vi "Thermocouple_Volts to Temperature.vi"(5 "Temperature Units":u16(ring) items=["Celsius", "Fahrenheit", "Kelvin", "Rankine"], 6 "ThermocoupleType":u16(ring)=2 items=["B", "E", "J", "K", "R", "S", "T", "N"], 7 "Thermocouple Voltage":sgl format="%.6f") -> (3 "Temperature":sgl format="%.6f")   [LabVIEW 2019]
doc: "Converts a voltage read from a thermocouple into a temperature.\n\nNational Instruments has chosen thermocouple polynomial expressions that are valid only for particular temperature ranges (given in the VI diagram). These polynomials come from the NIST Monograph 175.\n\nIf you wish to use a different conversion formula, you can edit this VI and enter your own equation into the appropriate formula node."
panel:
  # "Convert a thermocouple voltage\nto temperature."
  # "National Instruments has chosen thermocouple polynomial expressions that are valid only for  particular temperature ranges (given in the VI diagram).  These polynomials come from the NIST Monograph 175.\n\nIf you wish to use a different conversion formula, you can edit this VI and enter your own equation into the appropriate formula node."
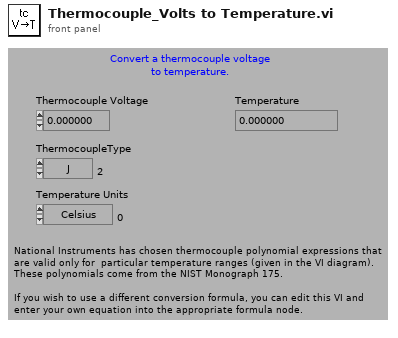
[diagram p1: front panel]
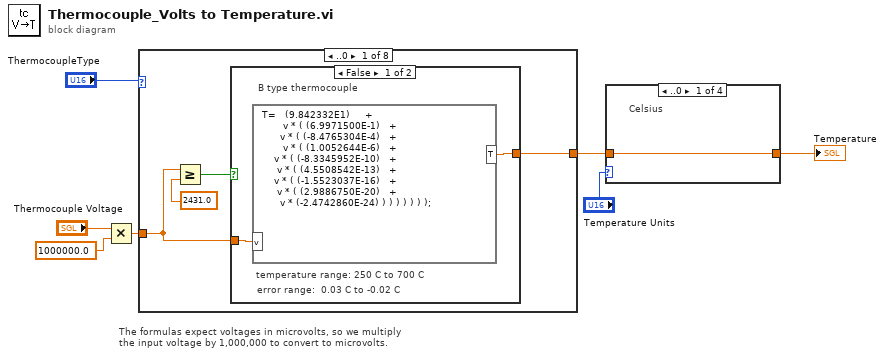
[diagram p0: block diagram]
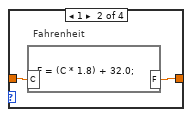
[diagram p2: hidden frame]
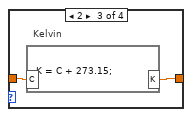
[diagram p3: hidden frame]
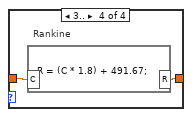
[diagram p4: hidden frame]
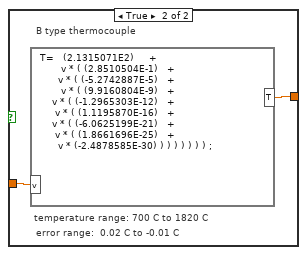
[diagram p5: hidden frame]
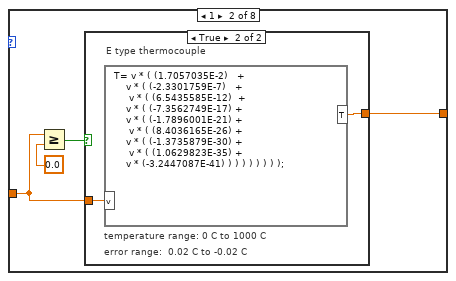
[diagram p6: hidden frame]
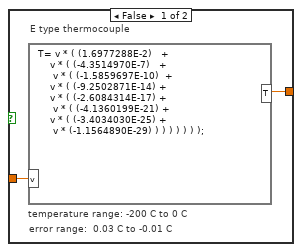
[diagram p7: hidden frame]
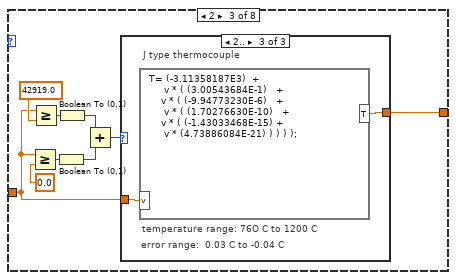
[diagram p8: hidden frame]
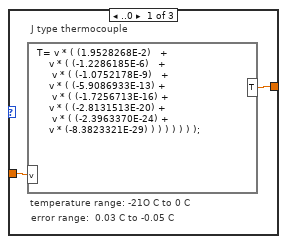
[diagram p9: hidden frame]
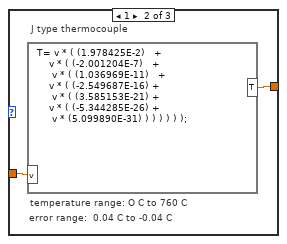
[diagram p10: hidden frame]
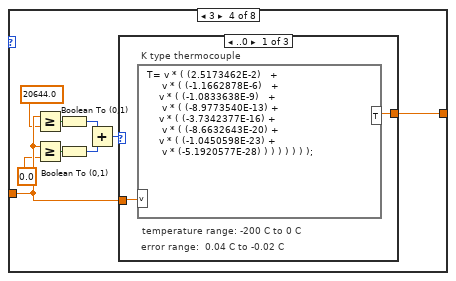
[diagram p11: hidden frame]
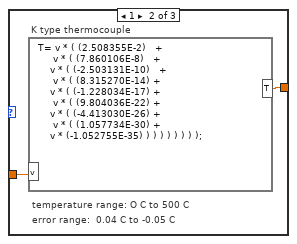
[diagram p12: hidden frame]
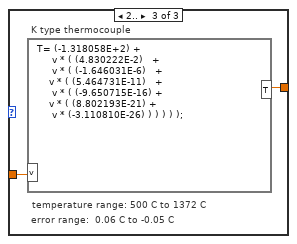
[diagram p13: hidden frame]
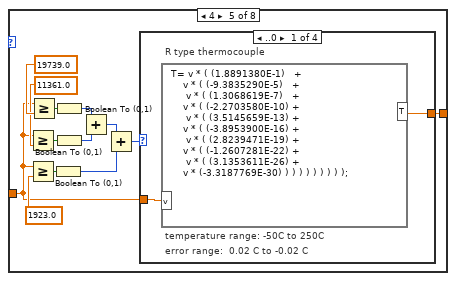
[diagram p14: hidden frame]
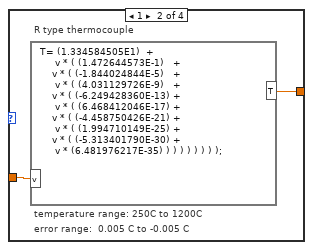
[diagram p15: hidden frame]
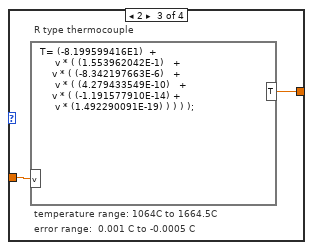
[diagram p16: hidden frame]
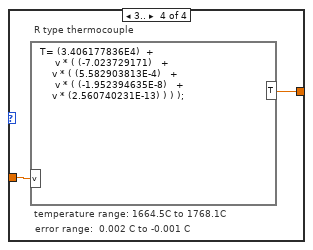
[diagram p17: hidden frame]
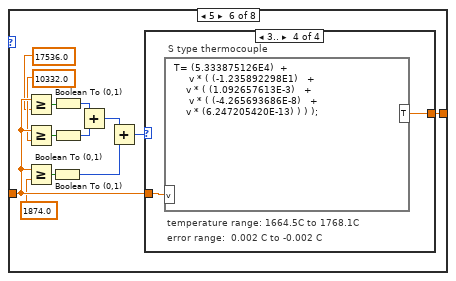
[diagram p18: hidden frame]
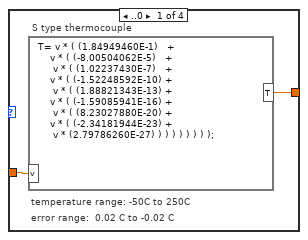
[diagram p19: hidden frame]
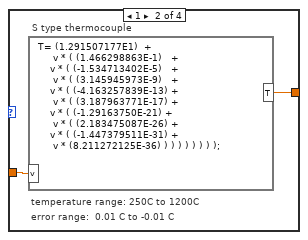
[diagram p20: hidden frame]
diagram:
  # "The formulas expect voltages in microvolts, so we multiply\nthe input voltage by 1,000,000 to convert to microvolts."
  n1 = Multiply(x="Thermocouple Voltage", y=sgl 1000000.0) -> (x*y=w4:sgl)
  n2 = case shown="..0" "ThermocoupleType" {
    tunnel: [w11 w18 w32 w39 w66 w87 w99 w111] -> w2
    tunnel: w4 -> [w9 w16 w24 w47 w54 w83 w96 w110]
    frame ..0 {
      n3 = Greater Or Equal?(x=w9, y=sgl 2431.0) -> (x >= y?=w10:bool)
      n4 = case shown="False" w10 {
        tunnel: w9 -> [w13 w15]
        tunnel: [w12 w14] -> w11
        frame False {
          # "error range:  0.03 C to -0.02 C"
          # "temperature range: 250 C to 700 C"
          # "B type thermocouple"
          n5 = formula code="T=   (9.842332E1)     +\n       v * ( (6.9971500E-1)   +\n      v * ( (-8.4765304E-4)   +\n       v * ( (1.0052644E-6)   +\n    v * ( (-8.3345952E-10)   +\n     v * ( (4.5508542E-13)   +\n    v * ( (-1.5523037E-16)   +\n     v * ( (2.9886750E-20)   +               \n      v * (-2.4742860E-24) ) ) ) ) ) ) );"("v"=w13) -> ("T"=w12:dbl)
        }
        frame True {
          # "error range:  0.02 C to -0.01 C"
          # "temperature range: 700 C to 1820 C"
          # "B type thermocouple"
          n6 = formula code="T=   (2.1315071E2)     +\n       v * ( (2.8510504E-1)   +\n      v * ( (-5.2742887E-5)   +\n       v * ( (9.9160804E-9)   +\n    v * ( (-1.2965303E-12)   +\n     v * ( (1.1195870E-16)   +\n    v * ( (-6.0625199E-21)   +\n     v * ( (1.8661696E-25)   +               \n      v * (-2.4878585E-30) ) ) ) ) ) ) ) ;"("v"=w15) -> ("T"=w14:dbl)
        }
      }
    }
    frame 1 {
      n7 = Greater Or Equal?(x=w16, y=sgl 0.0) -> (x >= y?=w19:bool)
      n8 = case shown="True" w19 {
        tunnel: w16 -> [w21 w23]
        tunnel: [w20 w22] -> w18
        frame False {
          # "error range:  0.03 C to -0.01 C"
          # "E type thermocouple"
          # "temperature range: -200 C to 0 C"
          n9 = formula code="T= v * ( (1.6977288E-2)   +\n    v * ( (-4.3514970E-7)   +\n     v * ( (-1.5859697E-10)  +\n    v * ( (-9.2502871E-14) +\n    v * ( (-2.6084314E-17) +\n     v * ( (-4.1360199E-21) +\n    v * ( (-3.4034030E-25) +\n     v * (-1.1564890E-29) ) ) ) ) ) ) );"("v"=w21) -> ("T"=w20:dbl)
        }
        frame True {
          # "error range:  0.02 C to -0.02 C"
          # "E type thermocouple"
          # "temperature range: 0 C to 1000 C"
          n10 = formula code="T= v * ( (1.7057035E-2)   +\n    v * ( (-2.3301759E-7)   +\n     v * ( (6.5435585E-12)  +\n    v * ( (-7.3562749E-17) +\n    v * ( (-1.7896001E-21) +\n     v * ( (8.4036165E-26) +\n    v * ( (-1.3735879E-30) +\n     v * ( (1.0629823E-35) +               \n    v * (-3.2447087E-41) ) ) ) ) ) ) ) );"("v"=w23) -> ("T"=w22:dbl)
        }
      }
    }
    frame 2 {
      n11 = Greater Or Equal?(x=w24, y=sgl 0.0) -> (x >= y?=w30:bool)
      n12 = Greater Or Equal?(x=w24, y=sgl 42919.0) -> (x >= y?=w31:bool)
      n13 = Boolean To (0,1)(Boolean=w30) -> (0, 1=w28:i16)
      n14 = Boolean To (0,1)(Boolean=w31) -> (0, 1=w29:i16)
      n15 = Add(x=w29, y=w28) -> (x+y=w27:i16)
      n16 = case shown="2.." w27 {
        tunnel: w24 -> [w33 w35 w38]
        tunnel: [w34 w36 w37] -> w32
        frame ..0 {
          # "error range:  0.03 C to -0.05 C"
          # "temperature range: -21O C to 0 C"
          # "J type thermocouple"
          n17 = formula code="T= v * ( (1.9528268E-2)   +\n    v * ( (-1.2286185E-6)   +\n     v * ( (-1.0752178E-9)   +\n    v * ( (-5.9086933E-13) +\n     v * ( (-1.7256713E-16) +\n    v * ( (-2.8131513E-20) +\n     v * ( (-2.3963370E-24) +\n    v * (-8.3823321E-29) ) ) ) ) ) ) );"("v"=w33) -> ("T"=w34:dbl)
        }
        frame 1 {
          # "error range:  0.04 C to -0.04 C"
          # "temperature range: O C to 760 C"
          # "J type thermocouple"
          n18 = formula code="T= v * ( (1.978425E-2)   +\n    v * ( (-2.001204E-7)   +\n     v * ( (1.036969E-11)   +\n    v * ( (-2.549687E-16) +\n     v * ( (3.585153E-21) +\n    v * ( (-5.344285E-26) +\n     v * (5.099890E-31) ) ) ) ) ) );"("v"=w35) -> ("T"=w36:dbl)
        }
        frame 2.. {
          # "error range:  0.03 C to -0.04 C"
          # "temperature range: 76O C to 1200 C"
          # "J type thermocouple"
          n19 = formula code="T= (-3.11358187E3)  +\n     v * ( (3.00543684E-1)   +\n    v * ( (-9.94773230E-6)   +\n     v * ( (1.70276630E-10)   +\n    v * ( (-1.43033468E-15) +\n     v * (4.73886084E-21) ) ) ) );"("v"=w38) -> ("T"=w37:dbl)
        }
      }
    }
    frame 3 {
      n20 = Greater Or Equal?(x=w47, y=sgl 20644.0) -> (x >= y?=w44:bool)
      n21 = Greater Or Equal?(x=w47, y=sgl 0.0) -> (x >= y?=w43:bool)
      n22 = Boolean To (0,1)(Boolean=w44) -> (0, 1=w42:i16)
      n23 = Boolean To (0,1)(Boolean=w43) -> (0, 1=w41:i16)
      n24 = Add(x=w42, y=w41) -> (x+y=w40:i16)
      n25 = case shown="..0" w40 {
        tunnel: w47 -> [w48 w50 w53]
        tunnel: [w49 w51 w52] -> w39
        frame ..0 {
          # "error range:  0.04 C to -0.02 C"
          # "temperature range: -200 C to 0 C"
          # "K type thermocouple"
          n26 = formula code="T= v * ( (2.5173462E-2)   +\n     v * ( (-1.1662878E-6)   +\n    v * ( (-1.0833638E-9)   +\n     v * ( (-8.9773540E-13) +\n    v * ( (-3.7342377E-16) +\n     v * ( (-8.6632643E-20) +\n    v * ( (-1.0450598E-23) +\n     v * (-5.1920577E-28) ) ) ) ) ) ) );"("v"=w48) -> ("T"=w49:dbl)
        }
        frame 1 {
          # "error range:  0.04 C to -0.05 C"
          # "temperature range: O C to 500 C"
          # "K type thermocouple"
          n27 = formula code="T= v * ( (2.508355E-2)   +\n     v * ( (7.860106E-8)   +\n    v * ( (-2.503131E-10)   +\n     v * ( (8.315270E-14) +\n    v * ( (-1.228034E-17) +\n     v * ( (9.804036E-22) +\n    v * ( (-4.413030E-26) +\n     v * ( (1.057734E-30) +               \n    v * (-1.052755E-35) ) ) ) ) ) ) ) );"("v"=w50) -> ("T"=w51:dbl)
        }
        frame 2.. {
          # "error range:  0.06 C to -0.05 C"
          # "temperature range: 500 C to 1372 C"
          # "K type thermocouple"
          n28 = formula code="T= (-1.318058E+2) +\n     v * ( (4.830222E-2)   +\n     v * ( (-1.646031E-6)   +\n    v * ( (5.464731E-11)   +\n     v * ( (-9.650715E-16) +\n    v * ( (8.802193E-21) +\n     v * (-3.110810E-26) ) ) ) ) );"("v"=w53) -> ("T"=w52:dbl)
        }
      }
    }
    frame 4 {
      n29 = Greater Or Equal?(x=w54, y=sgl 11361.0) -> (x >= y?=w64:bool)
      n30 = Greater Or Equal?(x=w54, y=sgl 1923.0) -> (x >= y?=w65:bool)
      n31 = Greater Or Equal?(x=w54, y=sgl 19739.0) -> (x >= y?=w63:bool)
      n32 = Boolean To (0,1)(Boolean=w65) -> (0, 1=w59:i16)
      n33 = Boolean To (0,1)(Boolean=w63) -> (0, 1=w62:i16)
      n34 = Boolean To (0,1)(Boolean=w64) -> (0, 1=w61:i16)
      n35 = Add(x=w62, y=w61) -> (x+y=w60:i16)
      n36 = Add(x=w60, y=w59) -> (x+y=w58:i16)
      n37 = case shown="..0" w58 {
        tunnel: w54 -> [w68 w70 w72 w74]
        tunnel: [w67 w69 w71 w73] -> w66
        frame ..0 {
          # "error range:  0.02 C to -0.02 C"
          # "temperature range: -50C to 250C"
          # "R type thermocouple"
          n38 = formula code="T= v * ( (1.8891380E-1)   +\n    v * ( (-9.3835290E-5)   +\n     v * ( (1.3068619E-7)   +\n    v * ( (-2.2703580E-10) +\n     v * ( (3.5145659E-13) +\n    v * ( (-3.8953900E-16) +\n     v * ( (2.8239471E-19) +\n    v * ( (-1.2607281E-22) +               \n     v * ( (3.1353611E-26) +\n    v * (-3.3187769E-30) ) ) ) ) ) ) ) ) );"("v"=w68) -> ("T"=w67:dbl)
        }
        frame 1 {
          # "error range:  0.005 C to -0.005 C"
          # "temperature range: 250C to 1200C"
          # "R type thermocouple"
          n39 = formula code="T= (1.334584505E1)  +\n     v * ( (1.472644573E-1)   +\n    v * ( (-1.844024844E-5)   +\n     v * ( (4.031129726E-9)   +\n    v * ( (-6.249428360E-13) +\n     v * ( (6.468412046E-17) +\n    v * ( (-4.458750426E-21) +\n     v * ( (1.994710149E-25) +\n    v * ( (-5.313401790E-30) +               \n     v * (6.481976217E-35) ) ) ) ) ) ) ) );"("v"=w70) -> ("T"=w69:dbl)
        }
        frame 2 {
          # "error range:  0.001 C to -0.0005 C"
          # "temperature range: 1064C to 1664.5C"
          # "R type thermocouple"
          n40 = formula code="T= (-8.199599416E1)  +\n     v * ( (1.553962042E-1)   +\n    v * ( (-8.342197663E-6)   +\n     v * ( (4.279433549E-10)   +\n    v * ( (-1.191577910E-14) +\n     v * (1.492290091E-19) ) ) ) );"("v"=w72) -> ("T"=w71:dbl)
        }
        frame 3.. {
          # "error range:  0.002 C to -0.001 C"
          # "temperature range: 1664.5C to 1768.1C"
          # "R type thermocouple"
          n41 = formula code="T= (3.406177836E4)  +\n     v * ( (-7.023729171)   +\n    v * ( (5.582903813E-4)   +\n     v * ( (-1.952394635E-8)   +\n    v * (2.560740231E-13) ) ) );"("v"=w74) -> ("T"=w73:dbl)
        }
      }
    }
    frame 5 {
      n42 = Greater Or Equal?(x=w83, y=sgl 17536.0) -> (x >= y?=w86:bool)
      n43 = Greater Or Equal?(x=w83, y=sgl 10332.0) -> (x >= y?=w85:bool)
      n44 = Greater Or Equal?(x=w83, y=sgl 1874.0) -> (x >= y?=w84:bool)
      n45 = Boolean To (0,1)(Boolean=w84) -> (0, 1=w75:i16)
      n46 = Boolean To (0,1)(Boolean=w86) -> (0, 1=w79:i16)
      n47 = Boolean To (0,1)(Boolean=w85) -> (0, 1=w78:i16)
      n48 = Add(x=w79, y=w78) -> (x+y=w76:i16)
      n49 = Add(x=w76, y=w75) -> (x+y=w77:i16)
      n50 = case shown="3.." w77 {
        tunnel: [w89 w91 w93 w95] -> w87
        tunnel: w83 -> [w88 w90 w92 w94]
        frame ..0 {
          # "error range:  0.02 C to -0.02 C"
          # "temperature range: -50C to 250C"
          # "S type thermocouple"
          n51 = formula code="T= v * ( (1.84949460E-1)   +\n    v * ( (-8.00504062E-5)   +\n     v * ( (1.02237430E-7)   +\n    v * ( (-1.52248592E-10) +\n     v * ( (1.88821343E-13) +\n    v * ( (-1.59085941E-16) +\n     v * ( (8.23027880E-20) +\n    v * ( (-2.34181944E-23) +               \n     v * (2.79786260E-27) ) ) ) ) ) ) ) );"("v"=w88) -> ("T"=w89:dbl)
        }
        frame 1 {
          # "error range:  0.01 C to -0.01 C"
          # "temperature range: 250C to 1200C"
          # "S type thermocouple"
          n52 = formula code="T= (1.291507177E1)  +\n     v * ( (1.466298863E-1)   +\n    v * ( (-1.534713402E-5)   +\n     v * ( (3.145945973E-9)   +\n    v * ( (-4.163257839E-13) +\n     v * ( (3.187963771E-17) +\n    v * ( (-1.29163750E-21) +\n     v * ( (2.183475087E-26) +\n    v * ( (-1.447379511E-31) +               \n     v * (8.211272125E-36) ) ) ) ) ) ) ) );"("v"=w90) -> ("T"=w91:dbl)
        }
        frame 2 {
          # "error range:  0.0002 C to -0.0002 C"
          # "temperature range: 1064C to 1664.5C"
          # "S type thermocouple"
          n53 = formula code="T= (-8.087801117E1)  +\n     v * ( (1.621573104E-1)   +\n    v * ( (-8.536869453E-6)   +\n     v * ( (4.719686976E-10)   +\n    v * ( (-1.441693666E-14) +\n     v * (2.081618890E-19) ) ) ) );"("v"=w92) -> ("T"=w93:dbl)
        }
        frame 3.. {
          # "error range:  0.002 C to -0.002 C"
          # "temperature range: 1664.5C to 1768.1C"
          # "S type thermocouple"
          n54 = formula code="T= (5.333875126E4)  +\n     v * ( (-1.235892298E1)   +\n    v * ( (1.092657613E-3)   +\n     v * ( (-4.265693686E-8)   +\n    v * (6.247205420E-13) ) ) );"("v"=w94) -> ("T"=w95:dbl)
        }
      }
    }
    frame 6 {
      n55 = Greater Or Equal?(x=w96, y=sgl 0.0) -> (x >= y?=w98:bool)
      n56 = case shown="False" w98 {
        tunnel: [w101 w103] -> w99
        tunnel: w96 -> [w100 w102]
        frame False {
          # "error range:  0.04 C to -0.02 C"
          # "temperature range: -200C to 0C"
          # "T type thermocouple"
          n57 = formula code="T= v * ( (2.5949192E-2)   +\n    v * ( (-2.1316967E-7)   +\n     v * ( (7.9018692E-10)  +\n    v * ( (4.2527777E-13) +\n     v * ( (1.3304473E-16) +\n    v * ( (2.0241446E-20) + \n     v * (1.2668171E-24) ) ) ) ) ) );"("v"=w100) -> ("T"=w101:dbl)
        }
        frame True {
          # "error range:  0.03 C to -0.03 C"
          # "temperature range: OC to 400C"
          # "T type thermocouple"
          n58 = formula code="T= v * ( (2.592800E-2)   +\n    v * ( (-7.602961E-7)   +\n     v * ( (4.637791E-11)  +\n    v * ( (-2.165394E-15) +\n     v * ( (6.048144E-20) +\n    v * (-7.293422E-25) ) ) ) ) );"("v"=w102) -> ("T"=w103:dbl)
        }
      }
    }
    frame 7.. {
      n59 = Greater Or Equal?(x=w110, y=sgl 20613.0) -> (x >= y?=w107:bool)
      n60 = Greater Or Equal?(x=w110, y=sgl 0.0) -> (x >= y?=w108:bool)
      n61 = Boolean To (0,1)(Boolean=w108) -> (0, 1=w104:i16)
      n62 = Boolean To (0,1)(Boolean=w107) -> (0, 1=w105:i16)
      n63 = Add(x=w105, y=w104) -> (x+y=w106:i16)
      n64 = case shown="..0" w106 {
        tunnel: w110 -> [w113 w115 w117]
        tunnel: [w114 w116 w118] -> w111
        frame ..0 {
          # "error range:  0.03 C to -0.02 C"
          # "temperature range: -200 C to 0 C"
          # "N type thermocouple"
          n65 = formula code="T= v * ( (3.8436847E-2)   +\n     v * ( (1.1010485E-6)   +\n    v * ( (5.2229312E-9)   +\n     v * ( (7.2060525E-12) +\n    v * ( (5.8488586E-15) +\n     v * ( (2.7754916E-18) +\n    v * ( (7.7075166E-22) +\n     v * ( (1.1582665E-25) +\n     v * (7.3138868E-30) ) ) ) ) ) ) ) );"("v"=w113) -> ("T"=w114:dbl)
        }
        frame 1 {
          # "error range:  0.03 C to -0.02 C"
          # "temperature range: O C to 600 C"
          # "N type thermocouple"
          n66 = formula code="T= v * ( (3.86896E-2)   +\n     v * ( (-1.08267E-6)   +\n    v * ( (4.70205E-11)   +\n     v * ( (-2.12169E-18) +\n    v * ( (-1.17272E-19) +\n     v * ( (5.39280E-24) +\n    v * (-7.98156E-29) ) ) ) ) ) );"("v"=w115) -> ("T"=w116:dbl)
        }
        frame 2.. {
          # "error range:  0.02 C to -0.04 C"
          # "temperature range: 600 C to 1300 C"
          # "N type thermocouple"
          n67 = formula code="T= (1.972485E1) +\n     v * ( (3.300943E-2)   +\n     v * ( (-3.915159E-7)   +\n    v * ( (9.855391E-12)   +\n     v * ( (-1.274371E-16) +\n    v * (7.767022E-22) ) ) ) );"("v"=w117) -> ("T"=w118:dbl)
        }
      }
    }
  }
  n68 = case shown="..0" "Temperature Units" {
    tunnel: w2 -> [w119 w121 w123 w125]
    tunnel: [w119 w120 w122 w124] -> w1
    frame ..0 {
      # "Celsius"
    }
    frame 1 {
      # "Fahrenheit"
      n69 = formula code="F = (C * 1.8) + 32.0;"("C"=w121) -> ("F"=w120:dbl)
    }
    frame 2 {
      # "Kelvin"
      n70 = formula code="K = C + 273.15;"("C"=w123) -> ("K"=w122:dbl)
    }
    frame 3.. {
      # "Rankine"
      n71 = formula code="R = (C * 1.8) + 491.67;"("C"=w125) -> ("R"=w124:dbl)
    }
  }
  "Temperature" <- w1
